vi "FindAllDepsList.vi"(9 "Dependency List [] In":string[](array[string]), 10 "Current Deps to Check":string, 11 "Dependency Map":map{string, string[]}(c390)) -> (3 "Dependency List [] Out":string[](array[string]))   [LabVIEW 2019, in "Hawkeye.lvlib"]
uses:
  Hawkeye.lvlib
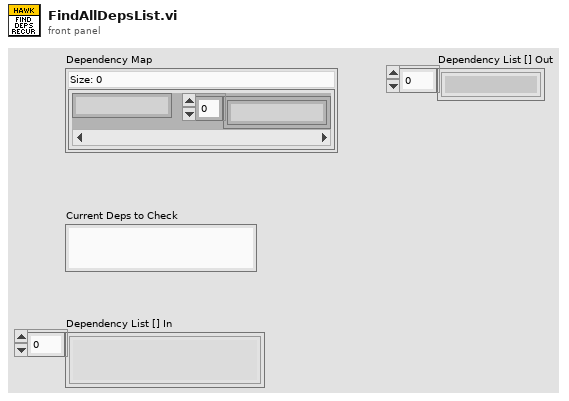
[diagram p1: front panel]
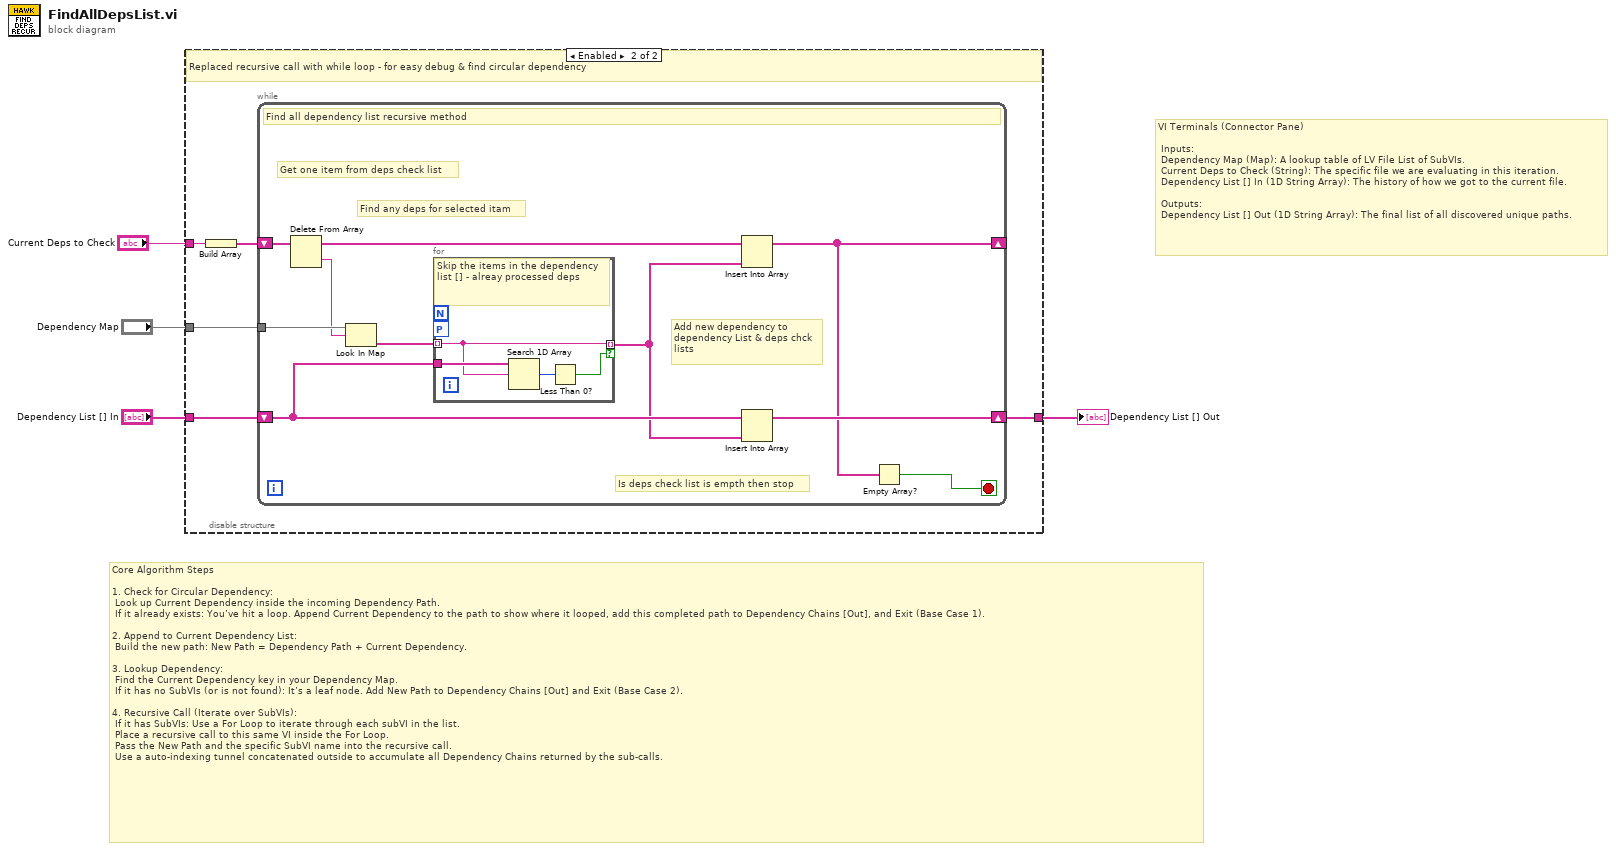
[diagram p0: block diagram]
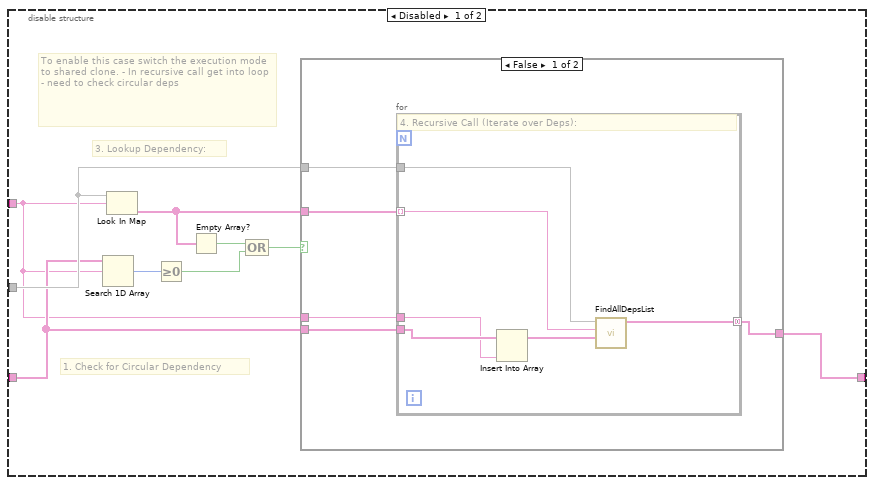
[diagram p2: hidden frame]
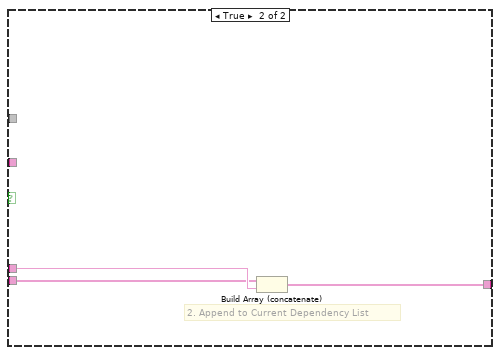
[diagram p3: hidden frame]
diagram:
  # "Core Algorithm Steps\n\n1. Check for Circular Dependency:\n Look up Current Dependency inside the incoming Dependency Path.\n If it already exists: You’ve hit a loop. Append Current Dependency to the path to show where it looped, add this completed path to Dependency Chains [Out], and Exit (Base Case 1).\n\n2. Append to Current Dependency List:\n Build the new path: New Path = Dependency Path + Current Dependency.\n\n3. Lookup Dependency:\n Find the Current Dependency key in your Dependency Map.\n If it has no SubVIs (or is not found): It’s a leaf node. Add New Path to Dependency Chains [Out] and Exit (Base Case 2).\n\n4. Recursive Call (Iterate over SubVIs):\n If it has SubVIs: Use a For Loop to iterate through each subVI in the list.\n Place a recursive call to this same VI inside the For Loop.\n Pass the New Path and the specific SubVI name into the recursive call.\n Use a auto-indexing tunnel concatenated outside to accumulate all Dependency Chains returned by the sub-calls."
  # "VI Terminals (Connector Pane)\n\n Inputs:\n Dependency Map (Map): A lookup table of LV File List of SubVIs.\n Current Deps to Check (String): The specific file we are evaluating in this iteration.\n Dependency List [] In (1D String Array): The history of how we got to the current file.\n\n Outputs:\n Dependency List [] Out (1D String Array): The final list of all discovered unique paths."
  n1 = disable-structure "Diagram Disable Structure" shown="Enabled" {
    disable-tunnel: [w12 w28] -> w4
    disable-tunnel: "Dependency Map" -> [w10 w32]
    disable-tunnel: "Dependency List [] In" -> [w8 w29]
    disable-tunnel: "Current Deps to Check" -> [w7 w31]
    frame Disabled {
      # "To enable this case switch the execution mode to shared clone. - In recursive call get into loop - need to check circular deps"
      # "3. Lookup Dependency:"
      # "1. Check for Circular Dependency"
      n2 = Search 1D Array(1D array=w8, element=w7) -> (index of element=w5:i32)  [unwired: 1 in]
      n3 = Look In Map(map=w10, key=w7) -> (value=w11:string[])  [unwired: 1 in, 1 out]
      n4 = Greater Or Equal To 0?(x=w5) -> (x >= 0?=w6:bool)
      n5 = Empty Array?(array=w11) -> (empty?=w13:bool)
      n6 = Compound Arithmetic op=OR(w13, w6) -> (w9:bool)
      n7 = case shown="False" w9 {
        tunnel: w10 -> [w18 _]
        tunnel: w11 -> [w17 _]
        tunnel: w7 -> [w16 w26]
        tunnel: w8 -> [w15 w25]
        tunnel: [w14 w27] -> w12
        frame False {
          n8 = for {
            tunnel: w18 -> [w24]
            tunnel: w17 -> [w23] mode=indexing
            tunnel: w16 -> [w19]
            tunnel: w15 -> [w21]
            tunnel: [w22] -> w14 mode=concatenating
            # "4. Recursive Call (Iterate over Deps):"
            n9 = Insert Into Array(array=w21, new element=w19) -> (w20:string[])  [unwired: 1 in]
            n10 = call "FindAllDepsList.vi"("Dependency List [] In"=w20, "Current Deps to Check"=w23, "Dependency Map"=w24) -> ("Dependency List [] Out"=w22:string[])  [unwired: 8 in]
          }
        }
        frame True {
          # "2. Append to Current Dependency List"
          n11 = Build Array (concatenate)(w25, w26) -> (w27:string[])
        }
      }
    }
    frame Enabled {
      # "Replaced recursive call with while loop - for easy debug & find circular dependency"
      n12 = Build Array(w31) -> (w30:string[])
      n13 = while {
        tunnel: w32 -> [w42]
        shift-right: [w34] -> _
        shift-left: w30 -> [w41]
        shift-right: [w36] -> w28
        shift-left: w29 -> [w37]
        stop <- w33 stop-if-true
        # "Is deps check list is empth then stop"
        # "Add new dependency to dependency List & deps chck lists"
        # "Find any deps for selected itam"
        # "Get one item from deps check list"
        # "Find all dependency list recursive method"
        n14 = Delete From Array "Delete From Array"(array=w41) -> (deleted portion=w40:string, array with subset deleted=w38:string[])  [unwired: 2 in]
        n15 = Look In Map(map=w42, key=w40) -> (value=w39:string[])  [unwired: 1 in, 1 out]
        n16 = for {
          tunnel: w39 -> [w45] mode=indexing
          tunnel: w37 -> [w46]
          tunnel: [w45] -> w35 mode=indexing if=w43
          workers-P: _ -> [_]
          # "Skip the items in the dependency list [] - alreay processed deps"
          n17 = Search 1D Array(1D array=w46, element=w45) -> (index of element=w44:i32)  [unwired: 1 in]
          n18 = Less Than 0?(x=w44) -> (x < 0?=w43:bool)
        }
        n19 = Insert Into Array(array=w38, new element=w35) -> (w34:string[])  [unwired: 1 in]
        n20 = Insert Into Array(array=w37, new element=w35) -> (w36:string[])  [unwired: 1 in]
        n21 = Empty Array?(array=w34) -> (empty?=w33:bool)
      }
    }
  }
  "Dependency List [] Out" <- w4
